vi "Page_Info_Update_Main_Destination_Name.vi"(8 "error in (no error)":errorcluster, 10 "destination name":string, 11 "AB_Build in":refnum<class "AB_Build.lvclass">) -> (0 "error out":errorcluster, 3 "AB_Build out":refnum<class "AB_Build.lvclass">)   [LabVIEW 2020, in "AB_Build.lvclass"]
uses:
  <vilib>/AppBuilder/AB_Classes/Build/AB_Build.lvclass
  <vilib>/AppBuilder/AB_Classes/Build/AB_Build.lvclass/AB_Build.ctl
  <vilib>/AppBuilder/AB_Classes/Destination/AB_Destination.lvclass
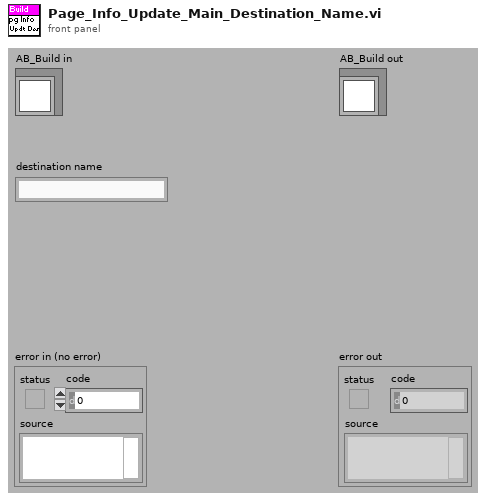
[diagram p1: front panel]
types:
  T1 = typedef "AB_Destination.ctl" = cluster{"destName":string, "path":path, "libraryName":string, "preserveHierarchy":bool, "eng_inBuild":bool, "eng_libraryReference":refnum<vi>, "eng_restictAddToNewLibrary":bool}
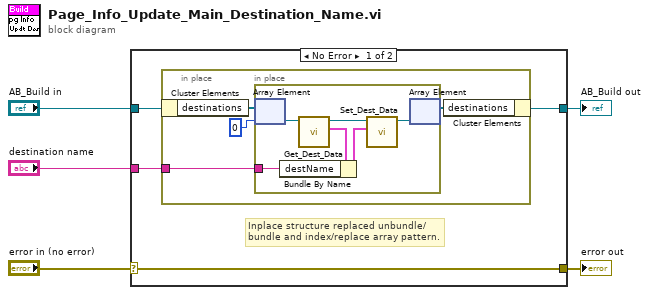
[diagram p0: block diagram]
diagram:
  n1 = case shown="No Error" "error in (no error)" {
    selector: "error in (no error)" -> [w9 w21]
    tunnel: [w9 w21] -> w4
    tunnel: [w7 w20] -> w2
    tunnel: "AB_Build in" -> [w8 w20]
    tunnel: "destination name" -> [w6 _]
    frame No Error {
      # "Inplace structure replaced unbundle/bundle and index/replace array pattern."
      n2 = in-place {
        in-place-border: w6 -> [w10]
        n3 = in-place-cluster #1(w8) -> ("destinations"=w13:refnum<class "AB_Destination.lvclass">[])
        n4 = in-place {
          in-place-border: w10 -> [w16]
          n5 = in-place-array #2(w13, 0) -> (w15:refnum<class "AB_Destination.lvclass">)
          n6 = call <vilib>:"Get_Dest_Data.vi"("Class in"=w15) -> ("destName"=w18:T1, "Class out"=w19:refnum<class "AB_Destination.lvclass">)  [unwired: 8 in, 1 out]
          n7 = Bundle By Name(cluster=w18, "destName"=w16) -> (w17:T1)
          n8 = call <vilib>:"Set_Dest_Data.vi"("destName"=w17, "Class in"=w19) -> ("Class out"=w14:refnum<class "AB_Destination.lvclass">)  [unwired: 8 in, 1 out]
          n9 = in-place-array #2(w14) -> (w11:refnum<class "AB_Destination.lvclass">[])  [unwired: 1 out]
        }
        n10 = in-place-cluster #1("destinations"=w11) -> (w7:refnum<class "AB_Build.lvclass">)
      }
    }
    frame Error {
    }
  }
  "error out" <- w4
  "AB_Build out" <- w2
